vi "Get Calibration path.vi"(8 "error in (no error)":errorcluster) -> (0 "error out":errorcluster, 2 "AO Cal Path":path, 3 "AI CAl Path":path)   [LabVIEW 2025]
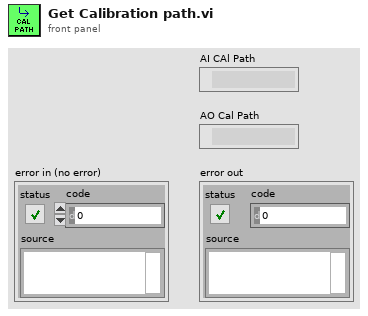
[diagram p1: front panel]
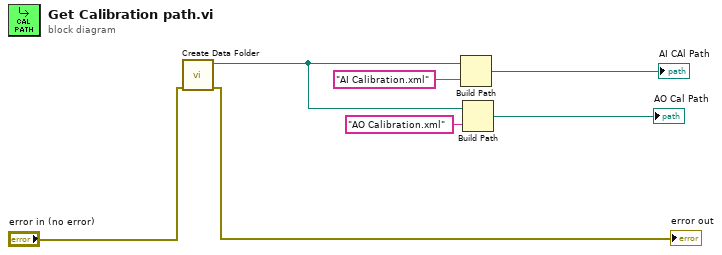
[diagram p0: block diagram]
diagram:
  n1 = call "Create Data Folder.vi"("error in (no error)"="error in (no error)") -> ("error out"=→"error out":errorcluster, "Data path"=w2:path)  [unwired: 9 in]
  n2 = Build Path(base path=w2, name or relative path="AI Calibration.xml") -> (appended path=→"AI CAl Path":path)
  n3 = Build Path(base path=w2, name or relative path="AO Calibration.xml") -> (appended path=→"AO Cal Path":path)
